vi "Slope Spacing and Counting Roughness.vi"(2 "Data":dbl[](array[numeric]), 3 "dx (1)":dbl=1.0) -> (5 "Rdq":dbl, 6 "Rda":dbl)   [LabVIEW 2018]
uses:
  <vilib>/Analysis/baseanly.llb/Mean (DBL).vi
  <vilib>/Analysis/5stat.llb/RMS (DBL).vi
  <vilib>/Analysis/NI_AALPro.lvlib
  <vilib>/Analysis/NI_AALBase.lvlib
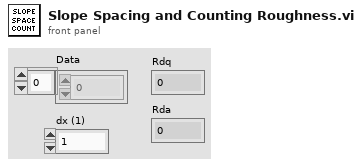
[diagram p1: front panel]
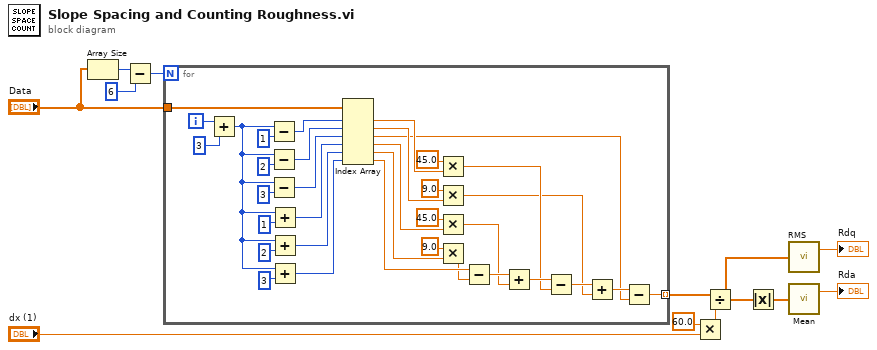
[diagram p0: block diagram]
diagram:
  n1 = Array Size(array="Data") -> (size(s)=w11:i32)
  n2 = Subtract(x=w11, y=6) -> (x-y=w12:i32)
  n3 = for {
    N: w12 -> [_]
    tunnel: "Data" -> [w47]
    tunnel: [w13] -> w8 mode=indexing
    i -> [w46]
    n4 = Add(x=w46, y=3) -> (x+y=w38:i32)
    n5 = Subtract(x=w38, y=1) -> (x-y=w37:i32)
    n6 = Subtract(x=w38, y=2) -> (x-y=w36:i32)
    n7 = Subtract(x=w38, y=3) -> (x-y=w35:i32)
    n8 = Add(x=w38, y=1) -> (x+y=w34:i32)
    n9 = Add(x=w38, y=2) -> (x+y=w33:i32)
    n10 = Add(x=w38, y=3) -> (x+y=w32:i32)
    n11 = Index Array(array=w47, index #1=w37, index #2=w36, index #3=w35, index #4=w34, index #5=w33, index #6=w32) -> (element #1=w24:dbl, element #2=w25:dbl, element #3=w14:dbl, element #4=w28:dbl, element #5=w30:dbl, element #6=w31:dbl)
    n12 = Multiply(x=45.0, y=w24) -> (x*y=w18:dbl)
    n13 = Multiply(x=9.0, y=w25) -> (x*y=w16:dbl)
    n14 = Multiply(x=45.0, y=w28) -> (x*y=w20:dbl)
    n15 = Multiply(x=9.0, y=w30) -> (x*y=w22:dbl)
    n16 = Subtract(x=w31, y=w22) -> (x-y=w21:dbl)
    n17 = Add(x=w21, y=w20) -> (x+y=w19:dbl)
    n18 = Subtract(x=w19, y=w18) -> (x-y=w17:dbl)
    n19 = Add(x=w17, y=w16) -> (x+y=w15:dbl)
    n20 = Subtract(x=w15, y=w14) -> (x-y=w13:dbl)
  }
  n21 = Multiply(x=60.0, y="dx (1)") -> (x*y=w7:dbl)
  n22 = Divide(x=w8, y=w7) -> (x/y=w3:dbl[])
  n23 = Absolute Value(x=w3) -> (abs(x)=w2:dbl[])
  n24 = call-poly <vilib>:"RMS.vi"("X"=w3) -> ("rms value"=→"Rdq":dbl)  [unwired: 1 out]
  n25 = call-poly <vilib>:"Mean.vi"("X"=w2) -> ("mean"=→"Rda":dbl)  [unwired: 1 out]
